vi "Set Sequence Line.vi"(8 "error in (no error)":errorcluster, 10 "Sequence Line":bool[](array[boolean]), 11 "VISA resource name":refnum<visa-resource-name>) -> (0 "error out":errorcluster, 3 "VISA resource name out":refnum<visa-resource-name>)   [LabVIEW 2020, in "QuPMXdriver.lvlib"]
doc: "Enable/disable multiple channels based on a 1D array of booleans. The array address channels in following matter: slave 1 channel 1; slave 1 channel 2; slave 2 channel 1, slave 2 channel 2, slave 3 channel 1 ..."
uses:
  QuPMXdriver.lvlib
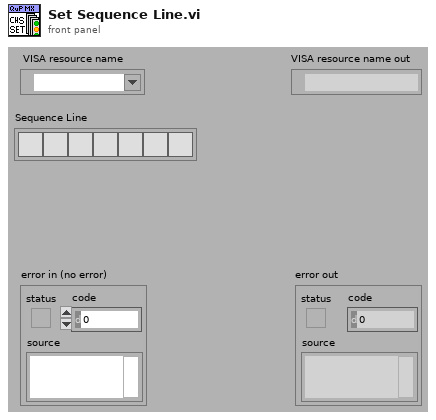
[diagram p1: front panel]
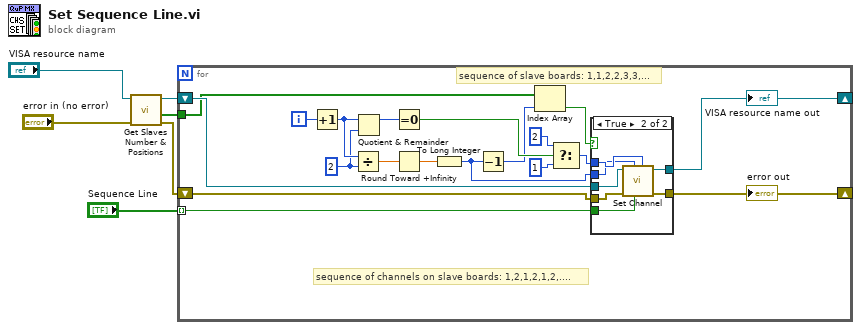
[diagram p0: block diagram]
diagram:
  n1 = call "Get Slaves Number & Positions.vi"("error in (no error)"="error in (no error)", "VISA resource name"="VISA resource name") -> ("error out"=w2:errorcluster, "Connected Slaves"=w7:bool[], "VISA resource name out"=w4:refnum<visa-resource-name>)  [unwired: 6 in, 1 out]
  n2 = for {
    tunnel: "Sequence Line" -> [w19] mode=indexing
    tunnel: w7 -> [w18]
    shift-right: [w23] -> w6
    shift-left: w4 -> [w22]
    shift-right: [w21] -> w1
    shift-left: w2 -> [w20]
    i -> [w17]
    w26 = 2 ("y")
    # "sequence of channels on slave boards: 1,2,1,2,1,2,...."
    # "sequence of slave boards: 1,1,2,2,3,3,..."
    n3 = Increment(x=w17) -> (x+1=w27:i32)
    n4 = Divide(x=w27, y=w26) -> (x/y=w25:dbl)
    n5 = Quotient & Remainder(x=w27, y=w26) -> (x-y*floor(x/y)=w14:i32)  [unwired: 1 out]
    n6 = Equal To 0?(x=w14) -> (x = 0?=w15:bool)
    n7 = Round Toward +Infinity(x=w25) -> (ceil(x): smallest int >= x=w24:dbl)
    n8 = To Long Integer(number=w24) -> (32bit integer=w10:i32)
    n9 = Decrement(x=w10) -> (x-1=w9:i32)
    n10 = Index Array(array=w18, index=w9) -> (element=w16:bool)
    n11 = Select(t=2 ("y"), s=w15, f=1 ("y")) -> (s? t:f=w11:i32)
    n12 = case shown="True" w16 {
      tunnel: w11 -> [_ w36]
      tunnel: w10 -> [_ w35]
      tunnel: [w29 w34] -> w23
      tunnel: w22 -> [w29 w33]
      tunnel: [w28 w32] -> w21
      tunnel: w20 -> [w28 w31]
      tunnel: w19 -> [_ w30]
      frame False {
      }
      frame True {
        n13 = call "Set Channel.vi"("Channel"=w36, "Channel Status"=w30, "Slave"=w35, "error in (no error)"=w31, "VISA resource name"=w33) -> ("error out"=w32:errorcluster, "VISA resource name out"=w34:refnum<visa-resource-name>)  [unwired: 5 in]
      }
    }
  }
  "error out" <- w1
  "VISA resource name out" <- w6
